vi "RP-VOA CONVERSION P to V.vi"(1 "Calibration points":dbl[](array[numeric]), 2 "% power":dbl) -> (0 "DAC Voltage":dbl)   [LabVIEW 2021]
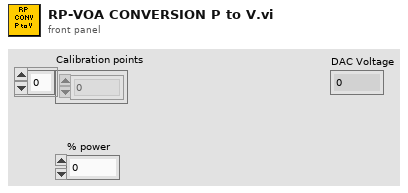
[diagram p1: front panel]
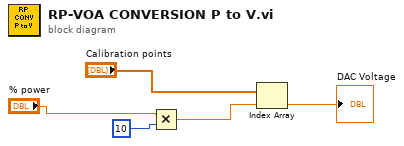
[diagram p0: block diagram]
diagram:
  n1 = Multiply(x="% power", y=10) -> (x*y=w1:dbl)
  n2 = Index Array(array="Calibration points", index=w1) -> (element=→"DAC Voltage":dbl)
